vi "Read Labels.vi"(8 "error in (no error)":errorcluster, 11 "Double Scanner in":refnum<class "Double Scanner.lvclass">) -> (0 "error out":errorcluster, 2 "Axis Label and Unit":T1[](array[typedef]), 3 "Double Scanner out":refnum<class "Double Scanner.lvclass">)   [LabVIEW 2023, in "Double Scanner.lvclass"]
uses:
  Double Scanner.lvclass
  Instruments/Utility Classes/Readable/Data Channel.ctl
  Instruments/Utility Classes/Readable/Data Point.ctl
  Instruments/Utility Classes/Readable/Time.ctl
  Instruments/Utility Classes/Readable/X.ctl
  Scanner/Scanner.lvclass
  Instruments/Utility Classes/Readable/Readable.lvclass
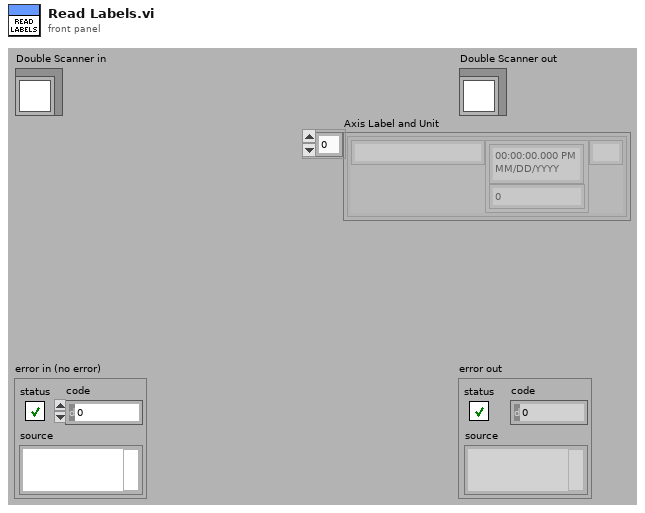
[diagram p1: front panel]
types:
  T1 = typedef "Readable.lvclass/Data Channel.ctl" = cluster{"Name":string, "Data Point":T2, "Unit":string}
  T2 = typedef "Readable.lvclass/Data Point.ctl" = cluster{"t":T3, "x":T4}
  T3 = typedef "Readable.lvclass/Time.ctl" = timestamp
  T4 = typedef "Readable.lvclass/X.ctl" = dbl
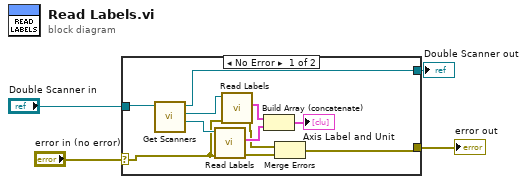
[diagram p0: block diagram]
diagram:
  n1 = case shown="No Error" "error in (no error)" {
    selector: "error in (no error)" -> [w8 w17]
    tunnel: [w5 w17] -> w3
    tunnel: "Double Scanner in" -> [w15 w16]
    tunnel: [w14 w16] -> w1
    frame No Error {
      n2 = call-dynamic "Get Scanners.vi"("Double Scanner in"=w15) -> ("Scanner 2 out"=w12:refnum<class "Scanner.lvclass">, "Scanner 1 out"=w13:refnum<class "Scanner.lvclass">, "Double Scanner out"=w14:refnum<class "Double Scanner.lvclass">)  [unwired: 7 in, 1 out]
      n3 = call-dynamic "Read Labels.vi"("error in (no error)"=w8, "Scanner in"=w12) -> ("error out"=w6:errorcluster, "Axis Label and Unit"=w10:T1[])  [unwired: 7 in, 1 out]
      n4 = call-dynamic "Read Labels.vi"("error in (no error)"=w8, "Scanner in"=w13) -> ("error out"=w7:errorcluster, "Axis Label and Unit"=w11:T1[])  [unwired: 7 in, 1 out]
      n5 = Build Array (concatenate)(w11, w10) -> (→"Axis Label and Unit":T1[])
      n6 = Merge Errors(w7, w6) -> (w5:errorcluster)
    }
    frame Error {
    }
  }
  "error out" <- w3
  "Double Scanner out" <- w1
